vi "DigitalInOut_input.vi"(8 "error in (no error)":errorcluster, 11 "DigitalInOut in":refnum<class "DigitalInOut.lvclass">) -> (0 "error out":errorcluster, 3 "DigitalInOut out":refnum<class "DigitalInOut.lvclass">)   [LabVIEW 2011, in "mbed_LVLibrary.lvlib" / "DigitalInOut.lvclass"]
uses:
  DigitalInOut.lvclass
  DigitalInOut.lvclass/DigitalInOut.ctl
  Transport Mechanisms/mbed/mbed.lvclass
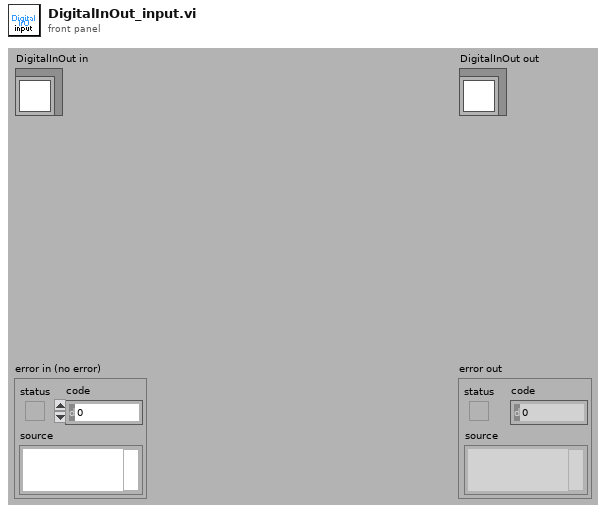
[diagram p1: front panel]
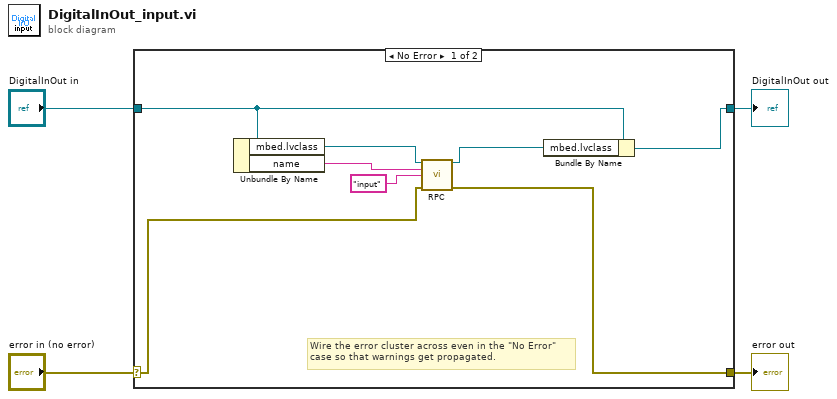
[diagram p0: block diagram]
diagram:
  n1 = case shown="No Error" "error in (no error)" {
    selector: "error in (no error)" -> [w6 w14]
    tunnel: [w5 w14] -> w3
    tunnel: [w12 w13] -> w1
    tunnel: "DigitalInOut in" -> [w11 w13]
    frame No Error {
      # "Wire the error cluster across even in the \"No Error\"\ncase so that warnings get propagated."
      n2 = Unbundle By Name(w11) -> ("mbed.lvclass"=w10:refnum<class "mbed.lvclass">, "name"=w8:string)
      n3 = call-dynamic "RPC.vi"("mbed in"=w10, "Name"=w8, "method"="input", "error in (no error)"=w6) -> ("mbed out"=w9:refnum<class "mbed.lvclass">, "error out"=w5:errorcluster)  [unwired: 9 in, 1 out]
      n4 = Bundle By Name(cluster=w11, "mbed.lvclass"=w9) -> (w12:refnum<class "DigitalInOut.lvclass">)
    }
    frame Error {
    }
  }
  "error out" <- w3
  "DigitalInOut out" <- w1
